vi "Calc Movement.vi"(8 "New Distance":dbl=1.0, 10 "Current":dbl=5.0 format="%#_13g", 11 "Desired":dbl=-10.0 format="%#_13g") -> (3 "New Current":dbl)   [LabVIEW 2022 SP3, in "MAS.lvlib" / "MAS ACTOR.lvclass"]
uses:
  MAS ACTOR.lvclass
panel:
  # "Connector Pane"
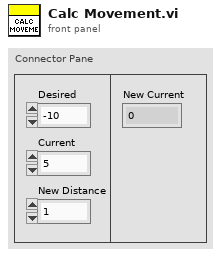
[diagram p1: front panel]
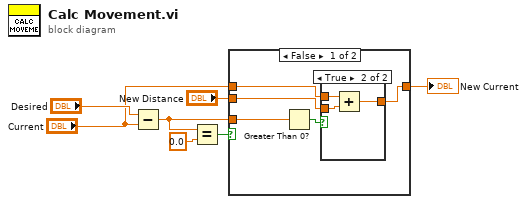
[diagram p0: block diagram]
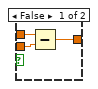
[diagram p2: hidden frame]
diagram:
  n1 = Subtract(x="Desired", y="Current") -> (x-y=w5:dbl)
  n2 = Equal?(x=w5, y=0.0) -> (x = y?=w7:bool)
  n3 = case shown="False" w7 {
    tunnel: "New Distance" -> [w12 _]
    tunnel: [w11 w19] -> w1
    tunnel: w5 -> [w9 _]
    tunnel: "Current" -> [w8 w19]
    frame False {
      n4 = Greater Than 0?(x=w9) -> (x > 0?=w10:bool)
      n5 = case shown="True" w10 {
        tunnel: w12 -> [w13 w18]
        tunnel: [w15 w17] -> w11
        tunnel: w8 -> [w14 w16]
        frame False {
          n6 = Subtract(x=w14, y=w13) -> (x-y=w15:dbl)
        }
        frame True {
          n7 = Add(x=w16, y=w18) -> (x+y=w17:dbl)
        }
      }
    }
    frame True {
    }
  }
  "New Current" <- w1
